vi "ADCMT7451A Read Single ADC.vi"() -> ()   [LabVIEW 2017]
doc: "This example shows how to configure a measurement and take a reading."
uses:
  Public/Configure/Configure DC Volts.vi
  Public/Configure/Configure AC Volts.vi
  Public/Configure/Configure DC Current.vi
  Public/Configure/Configure AC Current.vi
  Public/Configure/Configure 2W Resistance.vi
  Public/Configure/Configure 4W Resistance.vi
  ADCMT7451_ADC.lvlib
panel:
  in  "Function (0: DC Volts)":u16(ring) items=["DC Volts", "AC Volts", "DC Current", "AC Current", "2-Wire Resistance", "4-Wire Resistance"]
  out "Measurement":dbl
  in  "VISA resource name":refnum<visa-resource-name>
  # "(c) 2007 ADCMT ADC Corporation  ALL RIGHTS RESERVED."
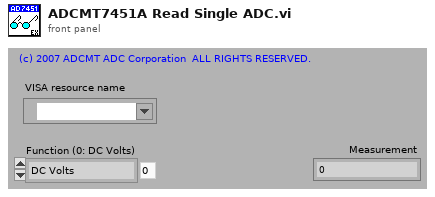
[diagram p1: front panel]
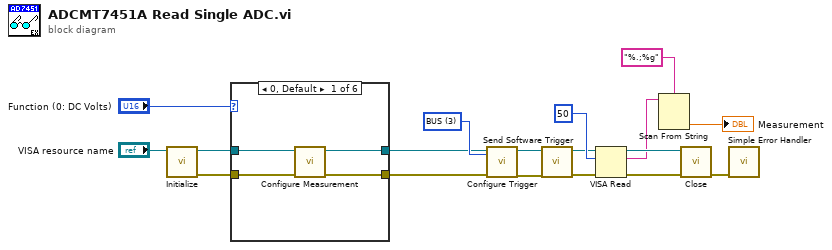
[diagram p0: block diagram]
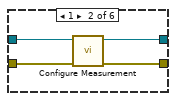
[diagram p2: hidden frame]
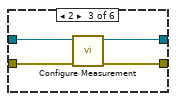
[diagram p3: hidden frame]
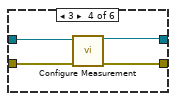
[diagram p4: hidden frame]
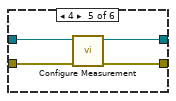
[diagram p5: hidden frame]
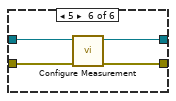
[diagram p6: hidden frame]
diagram:
  w6 = u16 3 items=["IMMEDIATE", "MANUAL", "EXTERNAL", "BUS", "LEVEL", "DELTA"]
  n1 = call "Initialize.vi"("VISA resource name"="VISA resource name") -> ("error out"=w12:errorcluster, "VISA resource name out"=w13:refnum<visa-resource-name>)  [unwired: 9 in]
  n2 = case shown="0, Default" "Function (0: DC Volts)" {
    tunnel: w13 -> [w22 w26 w28 w32 w38 w42]
    tunnel: [w19 w25 w29 w34 w37 w41] -> w5
    tunnel: [w20 w24 w30 w33 w36 w40] -> w7
    tunnel: w12 -> [w21 w23 w27 w31 w35 w39]
    frame 0, Default {
      n3 = call-poly "Configure Measurement.vi"("VISA resource name"=w22, "error in (no error)"=w21) -> ("VISA resource name out"=w19:refnum<visa-resource-name>, "error out"=w20:errorcluster)  [unwired: 16 in]
    }
    frame 1 {
      n4 = call-poly "Configure Measurement.vi"("VISA resource name"=w26, "error in (no error)"=w23) -> ("VISA resource name out"=w25:refnum<visa-resource-name>, "error out"=w24:errorcluster)  [unwired: 16 in]
    }
    frame 2 {
      n5 = call-poly "Configure Measurement.vi"("VISA resource name"=w28, "error in (no error)"=w27) -> ("VISA resource name out"=w29:refnum<visa-resource-name>, "error out"=w30:errorcluster)  [unwired: 16 in]
    }
    frame 3 {
      n6 = call-poly "Configure Measurement.vi"("VISA resource name"=w32, "error in (no error)"=w31) -> ("VISA resource name out"=w34:refnum<visa-resource-name>, "error out"=w33:errorcluster)  [unwired: 16 in]
    }
    frame 4 {
      n7 = call-poly "Configure Measurement.vi"("VISA resource name"=w38, "error in (no error)"=w35) -> ("VISA resource name out"=w37:refnum<visa-resource-name>, "error out"=w36:errorcluster)  [unwired: 16 in]
    }
    frame 5 {
      n8 = call-poly "Configure Measurement.vi"("VISA resource name"=w42, "error in (no error)"=w39) -> ("VISA resource name out"=w41:refnum<visa-resource-name>, "error out"=w40:errorcluster)  [unwired: 16 in]
    }
  }
  n9 = call "Configure Trigger.vi"("VISA resource name"=w5, "Trigger Source (0: Immediate)"=w6, "error in (no error)"=w7) -> ("VISA resource name out"=w2:refnum<visa-resource-name>, "error out"=w1:errorcluster)  [unwired: 15 in]
  n10 = call "Send Software Trigger.vi"("error in (no error)"=w1, "VISA resource name"=w2) -> ("error out"=w4:errorcluster, "VISA resource name out"=w3:refnum<visa-resource-name>)  [unwired: 8 in]
  n11 = VISA Read(VISA resource name=w3, byte count=50, error in (no error)=w4) -> (VISA resource name out=w16:refnum<visa-resource-name>, read buffer=w10:string, error out=w15:errorcluster)  [unwired: 1 out]
  n12 = Scan From String(format string="%.;%g", input string=w10) -> (output 1=→"Measurement":dbl)  [unwired: 3 in, 3 out]
  n13 = call "Close.vi"("error in (no error)"=w15, "VISA resource name"=w16) -> ("error out"=w18:errorcluster)  [unwired: 9 in]
  n14 = call <vilib>:"Simple Error Handler.vi"("error in (no error)"=w18) -> ()  [unwired: 4 in, 5 out]
